vi "ENPH 354 Assignment 3 - Q5.vi"() -> ()   [LabVIEW 2021]
uses:
  <vilib>/Utility/file.llb/Read Delimited Spreadsheet (string).vi
panel:
  out "Unscrambled\nMessage":string
  in  "Path":path
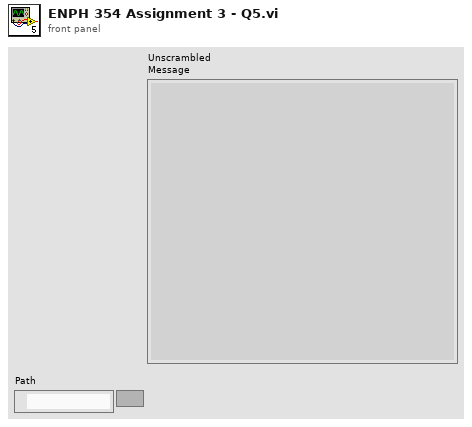
[diagram p1: front panel]
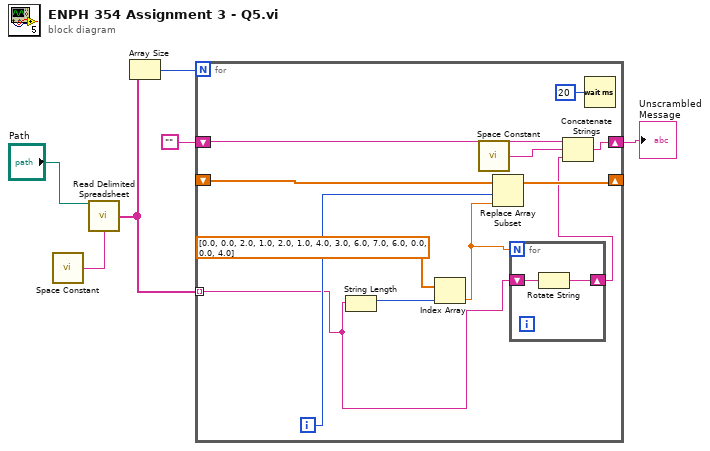
[diagram p0: block diagram]
diagram:
  n1 = call <vilib>:"Space Constant.vi"() -> ("String"=w1:string)
  n2 = call-poly <vilib>:"Read Delimited Spreadsheet.vi"("file path (dialog if empty)"="Path", "delimiter (\\t)"=w1) -> ("first row"=w5:string[])  [unwired: 8 in, 5 out]
  n3 = Array Size(array=w5) -> (size(s)=w2:i32)
  n4 = for {
    N: w2 -> [_]
    tunnel: w5 -> [w8] mode=indexing
    shift-right: [w11] -> w3
    shift-left: "" -> [w14]
    shift-right: [w15] -> _
    shift-left: _ -> [w16]
    i -> [w17]
    n5 = String Length(string=w8) -> (length=w18:i32)
    n6 = Index Array(array=dbl[] [0.0, 0.0, 2.0, 1.0, 2.0, 1.0, 4.0, 3.0, 6.0, 7.0, 6.0, 0.0, 0.0, 4.0], index=w18) -> (element=w7:dbl)
    n7 = call <vilib>:"Space Constant.vi"() -> ("String"=w12:string)
    n8 = Replace Array Subset(array=w16, new element=w7, index=w17) -> (w15:dbl[])
    n9 = for {
      N: w7 -> [_]
      shift-right: [w19] -> w13
      shift-left: w8 -> [w20]
      n10 = Rotate String(1:w20) -> (0:w19:string)
    }
    n11 = Concatenate Strings(w14, w12, w13) -> (w11:string)
    n12 = Wait (ms)(milliseconds to wait=u32 20) -> ()  [unwired: 1 out]
  }
  "Unscrambled\nMessage" <- w3
